vi "PathPlanner_PathPlanner_LoadPath.vi"(8 "Reversed":bool, 9 "MaxAcceleration":dbl, 10 "MaxVelocity":dbl, 11 "FileName":string="path1.path") -> (0 "error out":errorcluster, 2 "PathPlannerWayPoints":T7[](array[typedef]) {"HolonomicRotation"."SIN" format="%13.4f"; "HolonomicRotation"."COS" format="%13.4f"; "HolonomicRotation"."VALUE" format="%13.4f"; "NextControl"."Y" format="%14.3f"; "NextControl"."X" format="%14.3f"; "PrevControl"."Y" format="%14.3f"; "PrevControl"."X" format="%14.3f"; "AnchorPoint"."Y" format="%14.3f"; "AnchorPoint"."X" format="%14.3f"}, 3 "PathPlannerTrajectory":T1 {"States"."HolonomicAngular\nvelocity Deg/Sec"."SIN" format="%13.4f"; "States"."HolonomicAngular\nvelocity Deg/Sec"."COS" format="%13.4f"; "States"."HolonomicAngular\nvelocity Deg/Sec"."VALUE" format="%13.4f"; "States"."HolonomicRotation"."SIN" format="%13.4f"; "States"."HolonomicRotation"."COS" format="%13.4f"; "States"."HolonomicRotation"."VALUE" format="%13.4f"; "States"."AngularVelocity"."SIN" format="%13.4f"; "States"."AngularVelocity"."COS" format="%13.4f"; "States"."AngularVelocity"."VALUE" format="%13.4f"; "States"."TrajectoryState"."POSE"."ROTATION"."SIN" format="%13.4f"; "States"."TrajectoryState"."POSE"."ROTATION"."COS" format="%13.4f"; "States"."TrajectoryState"."POSE"."ROTATION"."VALUE" format="%13.4f"; "States"."TrajectoryState"."POSE"."TRANSLATION"."Y" format="%14.3f"; "States"."TrajectoryState"."POSE"."TRANSLATION"."X" format="%14.3f"; "States"."AngularAcceleration"."SIN" format="%13.4f"; "States"."AngularAcceleration"."COS" format="%13.4f"; "States"."AngularAcceleration"."VALUE" format="%13.4f"}, 4 "Full Filename":string)   [LabVIEW 2019, in "PathPlanner.lvlib"]
doc: "Load a path file from storage. This loads the waypoints from a file and calculates the trajectory states. It handles combining separate paths when reversal is flagged.\n\nInputs:\n - FileName -- The name of the path to load. Absolute or relative.\n - maxVel -- Max velocity of the path\n - maxAccel -- Max velocity of the path\n - reversed -- Should the robot follow the path reversed\n\nOutputs:\n - PathPlanner Trajectory -- The generated path (path planner trajectory) can be converted to trajectory)\n - Error -- error cluster\n\nNote:\n -- Default path for roboRIO is /home/lvuser/natinst/LabVIEW Data\n -- Default path for Windows is: %USERPROFILE%\\Documents\\LabVIEW Data"
uses:
  PathPlannerWaypoint.ctl
  <vilib>/Rock Robotics/WPI/ThirdParty/JAS_Junk/TrajLib/TypeDef/TRANSLATION2D.ctl
  <vilib>/Rock Robotics/WPI/ThirdParty/JAS_Junk/TrajLib/TypeDef/ROTATION2D.ctl
  PathPlannerTrajectory.ctl
  PathPlannerState.ctl
  <vilib>/Rock Robotics/WPI/ThirdParty/JAS_Junk/TrajLib/TypeDef/TRAJ_STATE.ctl
  <vilib>/Rock Robotics/WPI/ThirdParty/JAS_Junk/TrajLib/TypeDef/POSE2D.ctl
  PathPlanner.lvlib
  <vilib>/Rock Robotics/WPI/ThirdParty/JAS_Junk/TrajLib/Trajectory_Library.lvlib
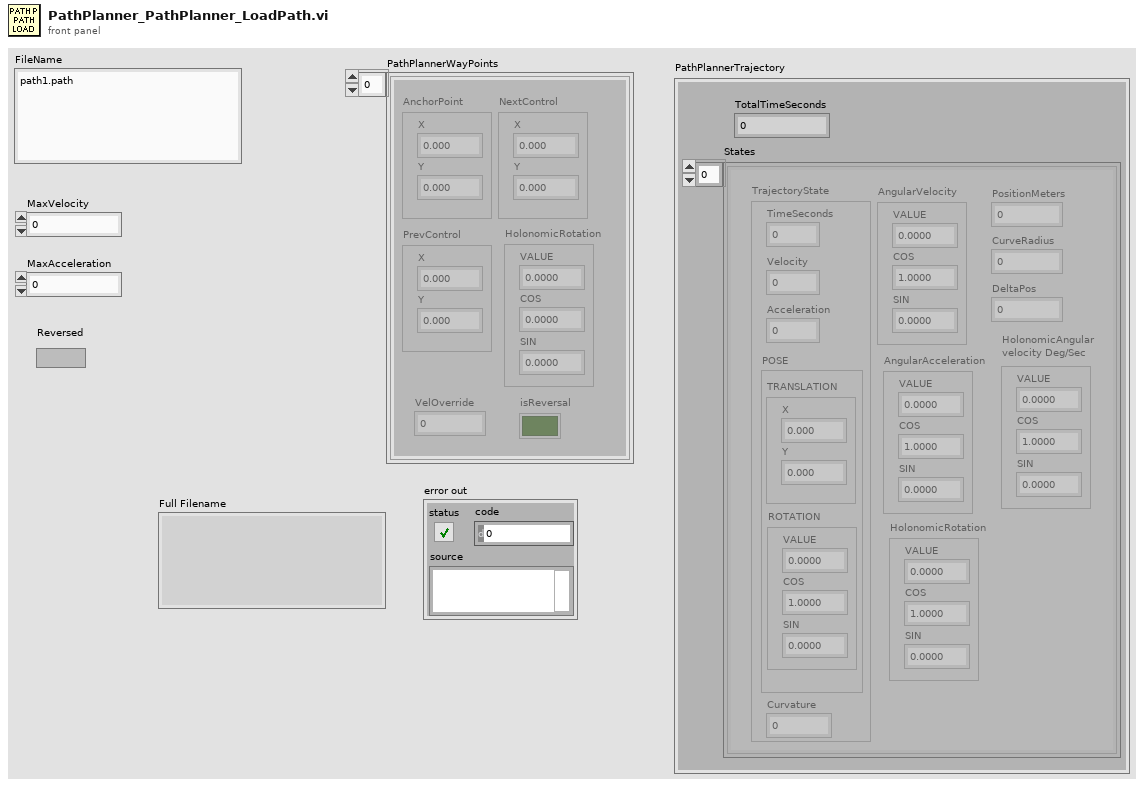
[diagram p1: front panel]
types:
  T1 = typedef "PathPlanner.lvlib/PathPlannerTrajectory.ctl" = cluster{"TotalTimeSeconds":dbl, "States":T2[]}
  T2 = typedef "PathPlanner.lvlib/PathPlannerState.ctl" = cluster{"AngularAcceleration":T3, "PositionMeters":dbl, "TrajectoryState":T4, "AngularVelocity":T3, "HolonomicRotation":T3, "CurveRadius":dbl, "DeltaPos":dbl, "HolonomicAngular\nvelocity Deg/Sec":T3}
  T3 = typedef "Trajectory_Library.lvlib/ROTATION2D.ctl" = cluster{"VALUE":dbl, "COS":dbl, "SIN":dbl}
  T4 = typedef "Trajectory_Library.lvlib/TRAJ_STATE.ctl" = cluster{"TimeSeconds":dbl, "Velocity":dbl, "Acceleration":dbl, "POSE":T5, "Curvature":dbl}
  T5 = typedef "Trajectory_Library.lvlib/POSE2D.ctl" = cluster{"TRANSLATION":T6, "ROTATION":T3}
  T6 = typedef "Trajectory_Library.lvlib/TRANSLATION2D.ctl" = cluster{"X":dbl, "Y":dbl}
  T7 = typedef "PathPlanner.lvlib/PathPlannerWaypoint.ctl" = cluster{"AnchorPoint":T6, "PrevControl":T6, "NextControl":T6, "HolonomicRotation":T3, "VelOverride":dbl, "isReversal":bool}
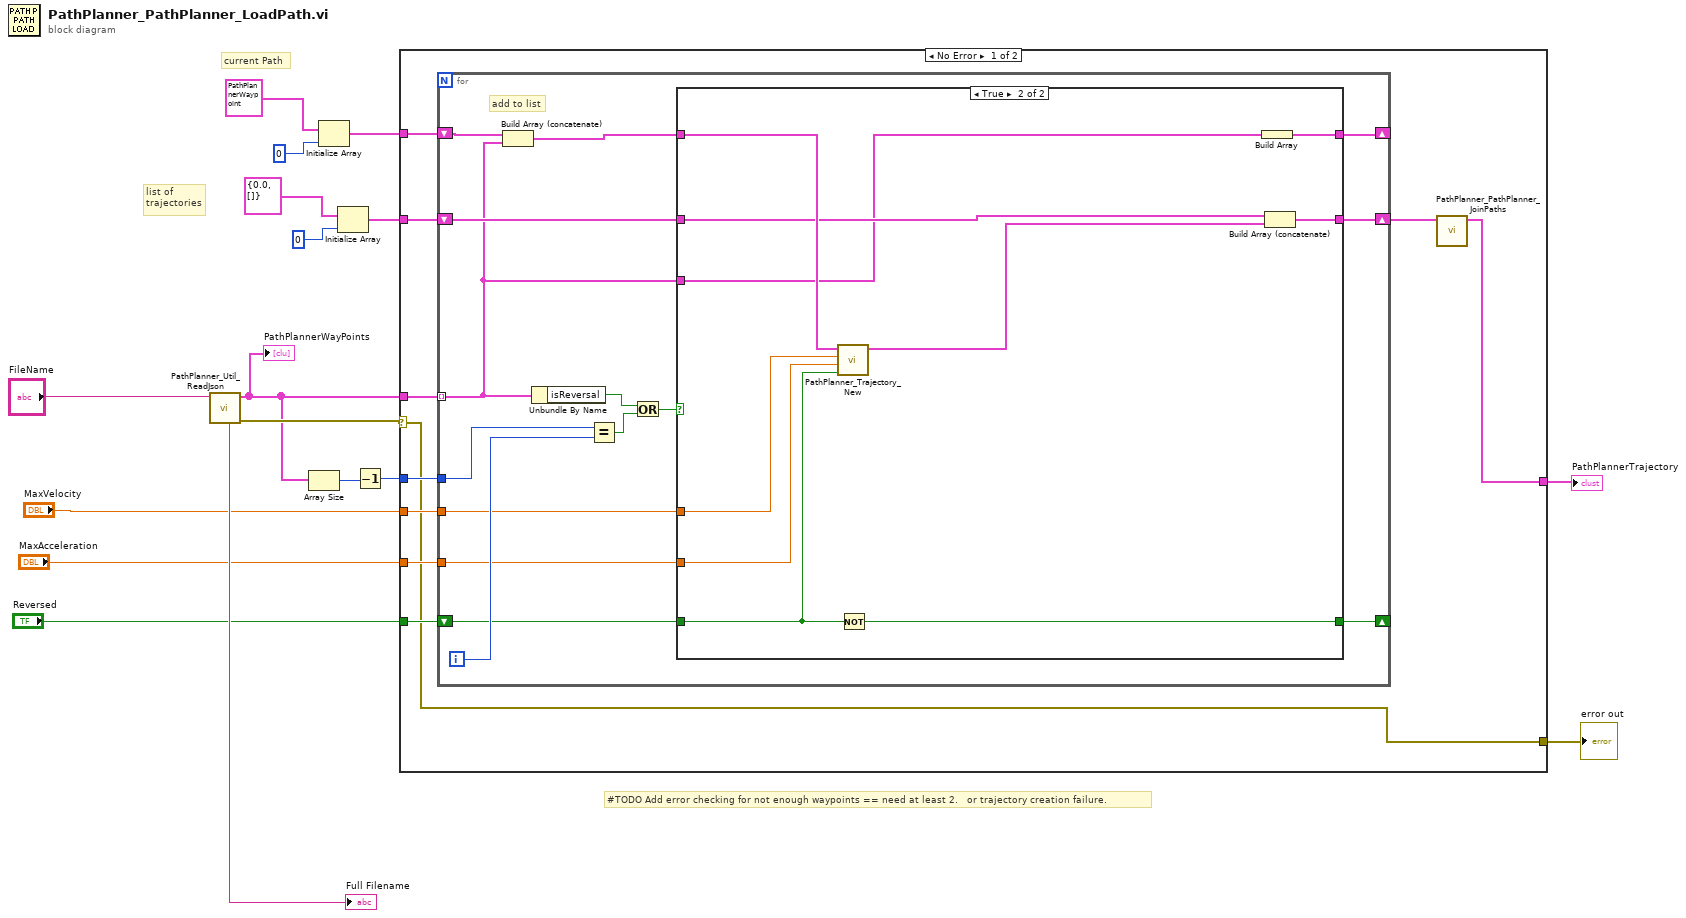
[diagram p0: block diagram]
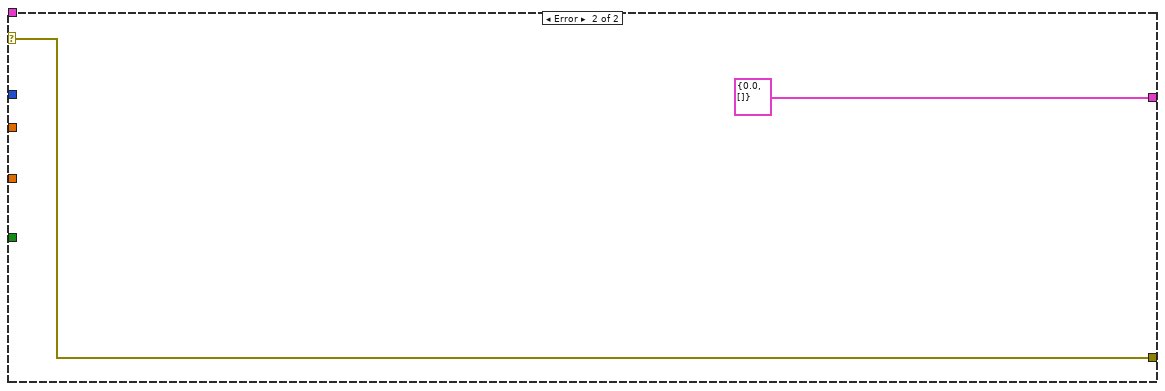
[diagram p3: hidden frame]
diagram:
  # "#TODO Add error checking for not enough waypoints == need at least 2.   or trajectory creation failure."
  # "list of \ntrajectories"
  # "current Path"
  n1 = call "PathPlanner_Util_ReadJson.vi"("FileName"="FileName") -> ("error out"=w15:errorcluster, "PathPlannerWayPoints"=w3:T7[], "Full Filename"=→"Full Filename":string)  [unwired: 8 in]
  "PathPlannerWayPoints" <- w3
  n2 = Array Size(array=w3) -> (size(s)=w9:i32)
  n3 = Initialize Array(T7 {"AnchorPoint"={"X"=0.0, "Y"=0.0}, "PrevControl"={"X"=0.0, "Y"=0.0}, "NextControl"={"X"=0.0, "Y"=0.0}, "HolonomicRotation"={"VALUE"=0.0, "COS"=1.0, "SIN"=0.0}, "VelOverride"=0.0, "isReversal"=FALSE} ("PathPlannerWaypoint"), 0 ("dimension size")) -> (w12:T7[])
  n4 = Initialize Array(T1 {"TotalTimeSeconds"=0.0, "States"=[]} ("PathPlannerTrajectory"), 0 ("dimension size")) -> (w7:T1[])
  n5 = Decrement(x=w9) -> (x-1=w8:i32)
  n6 = case shown="No Error" w15 {
    selector: w15 -> [w20 w56]
    tunnel: w12 -> [w27 _]
    tunnel: w3 -> [w26 _]
    tunnel: w8 -> [w25 _]
    tunnel: w7 -> [w24 _]
    tunnel: "MaxVelocity" -> [w23 _]
    tunnel: "MaxAcceleration" -> [w22 _]
    tunnel: "Reversed" -> [w21 _]
    tunnel: [w18 T1 {"TotalTimeSeconds"=0.0, "States"=[]} ("PathPlannerTrajectory")] -> w2
    tunnel: [w20 w56] -> w1
    frame No Error {
      n7 = for {
        shift-right: [w33] -> _
        shift-left: w27 -> [w42]
        tunnel: w26 -> [w28] mode=indexing
        tunnel: w25 -> [w39]
        shift-right: [w35] -> w19
        shift-left: w24 -> [w36]
        tunnel: w23 -> [w32]
        tunnel: w22 -> [w31]
        shift-right: [w29] -> _
        shift-left: w21 -> [w30]
        i -> [w38]
        # "add to list"
        n8 = Build Array (concatenate)(w42, w28) -> (w34:T7[])
        n9 = Unbundle By Name(w28) -> ("isReversal"=w41:bool)
        n10 = Equal?(x=w39, y=w38) -> (x = y?=w40:bool)
        n11 = Or(x=w41, y=w40) -> (x .or. y?=w37:bool)
        n12 = case shown="True" w37 {
          tunnel: w36 -> [w45 w51]
          tunnel: [w45 w52] -> w35
          tunnel: w34 -> [w44 w55]
          tunnel: [w44 w47] -> w33
          tunnel: w32 -> [_ w54]
          tunnel: w31 -> [_ w53]
          tunnel: w30 -> [w43 w48]
          tunnel: [w43 w49] -> w29
          tunnel: w28 -> [_ w46]
          frame False {
          }
          frame True {
            n13 = call "PathPlanner_Trajectory_New.vi"("Reversed"=w48, "MaxAccel"=w53, "MaxVelocity"=w54, "PathPoints"=w55) -> ("PathPlannerTrajectory"=w50:T1)  [unwired: 7 in]
            n14 = Not(x=w48) -> (.not. x?=w49:bool)
            n15 = Build Array(w46) -> (w47:T7[])
            n16 = Build Array (concatenate)(w51, w50) -> (w52:T1[])
          }
        }
      }
      n17 = call "PathPlanner_PathPlanner_JoinPaths.vi"("in Trajectories"=w19) -> ("out PathPlannerTrajectory"=w18:T1)  [unwired: 10 in]
    }
    frame Error {
    }
  }
  "error out" <- w1
  "PathPlannerTrajectory" <- w2
